vi "GetAlazar_SaveToFile_25_AVG.vi"(0 "AlazarCluster":T5, 1 "Digitizer Settings":T1={"Digitizer delay (us) "=0.0, "rf points per line"=2048, "lines per plane"=128, "Samp Rate (Hz)"=100000000.0, "Additional dig delay (us)"=0.0, "Voltage Scale"=0.4, "Pre-Looks"=0, "Offset delay (us)"=0.0, "bits A/D"=8, "Avg Num"=1, "DigTimeOut"=5.0, "Rel Dig Delay"=0.0, "Dig Ch"=0, "LeCroyCluster"={"LeCroy Channels"=[TRUE, FALSE, FALSE, FALSE], "LC read pt offset"=0.0, "Sweep Avg"=FALSE}, "Main Digitizer"=enum."NI Digitizer", "Dig Config"=enum."Single channel", "Digitizer ID Cluster"={"Acqiris/Alazar/SP ID"=[], "NI Instr Handles"=[], "LeCroy VISA"="", "GaGe Handle"={"Handle"=0, "Sample size"=0, "Resolution"=0, "Offset"=0, "Channels"=0, "Boards"=0}, "ATS Ref"="ATS9350", "Acqiris Address"=["PCI::INSTR0"], "ADQRef"=refnum, "adq_cu_ptr"=refnum}, "Trigger Settings"={"Trig Source"=1, "Trig Coupling"=0, "Trig Slope"=0, "Level (mV)"=1500.0}, "Bulk Acq"=FALSE, "Bulk Start Indexes"=[], "Data Ref RF"=refnum, "NI ID/Channel"=[], "Total Dig CH"=1, "Xtra Ann Trig delay (us)"=10.0, "Fix Z Delay?"=FALSE, "One Way Transmission?"=FALSE, "Data Ref Log"=refnum} {"Trigger Settings"."Trig Slope" items=["Positive", "Negative"]; "Trigger Settings"."Level (mV)" format="%.2f"; "Trigger Settings"."Trig Coupling" items=["DC 1 MOhm", "AC 1 MOhm", "DC 50 Ohm", "AC 50 Ohm"]; "Trigger Settings"."Trig Source" items=["Chan 1", "External"]; "Rel Dig Delay" format="%.2f"; "DigTimeOut" format="%.2f"; "Avg Num" min=1; "Offset delay (us)" format="%.2f"; "Additional dig delay (us)" format="%.2f"; "Digitizer delay (us)" format="%.2f"}, 7 "errorin":errorcluster, 8 "File Array":string[](array[string]), 10 "lines per plane":i32) -> (17 "Raw VGain (scale)":dbl, 18 "Gain Array":T6(array[cluster]), 20 "data out":i16[][][](array[numeric]), 21 "VGain (dB)":dbl, 27 "error out":errorcluster)   [LabVIEW 2022 SP3]
uses:
  -DigitizerRoutines/DigitizerSettings.ctl
  -DigitizerRoutines/DigitizerID.ctl
  -DigitizerRoutines/Digitizer.ctl
  -DigitizerRoutines/DigConfig.ctl
  C:/Windows/System32/ADQAPI_dotNet_helper.dll
panel:
  out "read time":u32
  out "save time":u32
  out "Numeric":i32
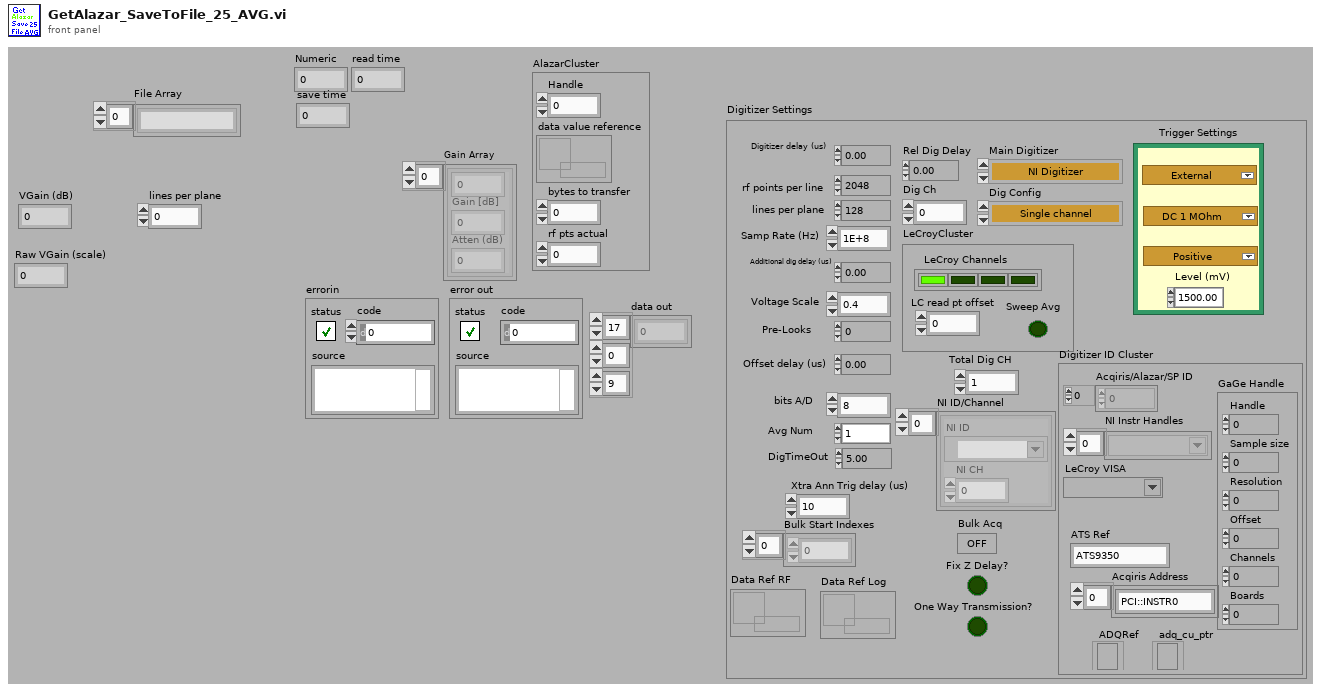
[diagram p1: front panel]
types:
  T1 = typedef "DigitizerSettings.ctl" = cluster{"Digitizer delay (us) ":dbl, "rf points per line":i32, "lines per plane":i32, "Samp Rate (Hz)":dbl, "Additional dig delay (us)":dbl, "Voltage Scale":dbl, "Pre-Looks":i32, "Offset delay (us)":dbl, "bits A/D":i8, "Avg Num":i32, "DigTimeOut":sgl, "Rel Dig Delay":sgl, "Dig Ch":i32, "LeCroyCluster":cluster{"LeCroy Channels":bool[], "LC read pt offset":dbl, "Sweep Avg":bool}, "Main Digitizer":T2, "Dig Config":T3, "Digitizer ID Cluster":T4, "Trigger Settings":cluster{"Trig Source":u16, "Trig Coupling":u16, "Trig Slope":u16, "Level (mV)":dbl}, "Bulk Acq":bool, "Bulk Start Indexes":i32[], "Data Ref RF":refnum<data-value>, "NI ID/Channel":cluster{"NI ID":refnum<k15>, "NI CH":i32}[], "Total Dig CH":i32, "Xtra Ann Trig delay (us)":dbl, "Fix Z Delay?":bool, "One Way Transmission?":bool, "Data Ref Log":refnum<data-value>}
  T2 = typedef "Digitizer.ctl" = enum16{"Acqiris Digitizer", "NI Digitizer", "LeCroy", "GaGe", "AlazarTech", "No Digitizer", "Teledyne"}
  T3 = typedef "DigConfig.ctl" = enum16{"Single channel", "2 Chans w/ 2 Acqiris", "2 Chans w/ 1 Acqiris", "5-CH Pulser New", "5-CH pulser w/ ann array", "5-pass style ann array", "Empty"}
  T4 = typedef "DigitizerID.ctl" = cluster{"Acqiris/Alazar/SP ID":u32[], "NI Instr Handles":refnum<k15>[], "LeCroy VISA":refnum<visa-resource-name>, "GaGe Handle":cluster{"Handle":u32, "Sample size":u32, "Resolution":i32, "Offset":i32, "Channels":u32, "Boards":u32}, "ATS Ref":string, "Acqiris Address":string[], "ADQRef":refnum<k24>, "adq_cu_ptr":refnum<k24>}
  T5 = cluster{"Handle":u32, "data value reference":refnum<data-value>, "bytes to transfer":u32, "rf pts actual":u32}
  T6 = cluster{sgl, "Gain [dB]  ":sgl, "Atten (dB)":sgl}[]
  T7 = cluster{"wfm":i16[][], "max queue size (-1, unlimited)":i32}
  T8 = cluster{sgl, "Gain [dB]  ":sgl, "Atten (dB)":sgl}
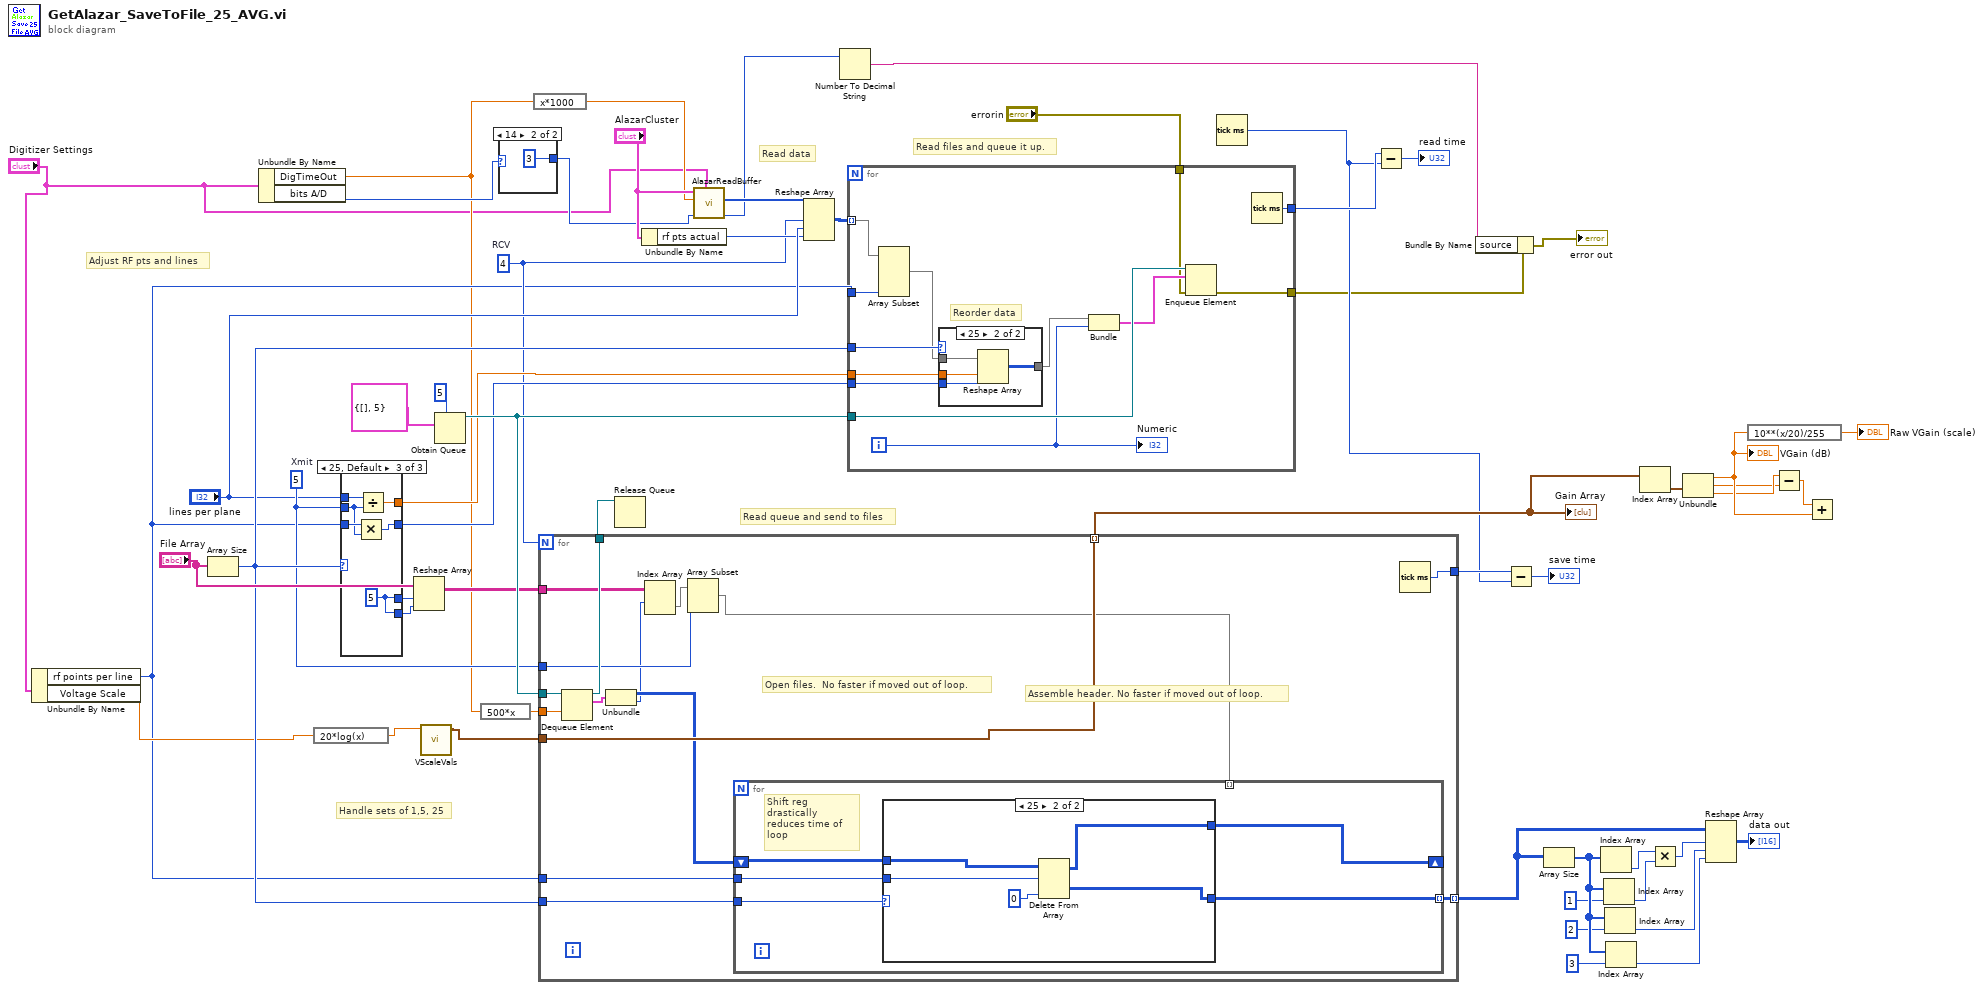
[diagram p0: block diagram]
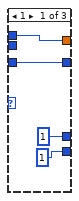
[diagram p4: hidden frame]
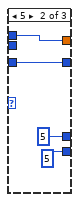
[diagram p5: hidden frame]
diagram:
  w30 = 5  # Xmit
  w24 = 4  # RCV
  # "Read data"
  # "Adjust RF pts and lines"
  # "Handle sets of 1,5, 25"
  # "Read files and queue it up."
  # "Read queue and send to files"
  n1 = Unbundle By Name("Digitizer Settings") -> ("rf points per line"=w4:i32, "Voltage Scale"=w5:dbl)
  n2 = Array Size(array="File Array") -> (size(s)=w34:i32)
  n3 = Unbundle By Name("Digitizer Settings") -> ("DigTimeOut"=w2:sgl, "bits A/D"=w3:i8)
  n4 = expression code="20*log(x)"(w5) -> (w32:dbl)
  n5 = case shown="25, Default" w34 {
    tunnel: [1 5 w70] -> w39
    tunnel: [w59 w63 w66] -> w36
    tunnel: w4 -> [w59 w63 w67]
    tunnel: [w58 w62 w68] -> w37
    tunnel: "lines per plane" -> [w58 w62 w69]
    tunnel: [1 5 w70] -> w38
    tunnel: w30 -> [_ _ w65]
    frame 1 {
    }
    frame 5 {
    }
    frame 25, Default {
      w70 = 5
      n6 = Multiply(x=w67, y=w65) -> (x*y=w66:i32)
      n7 = Divide(x=w69, y=w65) -> (x/y=w68:dbl)
    }
  }
  n8 = Reshape Array("File Array", w39, w38) -> (w33:string[][])
  n9 = call "VScaleVals.vi"("Full Scale"=w32) -> ("Voltage Scale"=w31:T8)  [unwired: 8 in, 2 out]
  n10 = Obtain Queue(max queue size (-1, unlimited)=5, element data type=T7 {"wfm"=[], "max queue size (-1, unlimited)"=5}) -> (queue out=w48:refnum<queue>)  [unwired: 3 in, 2 out]
  n11 = expression code="500*x"(w2) -> (w35:sgl)
  n12 = case shown="14" w3 {
    tunnel: [_ u16 3 ("Extra Shift")] -> w17
    frame 0, Default {
    }
    frame 14 {
    }
  }
  n13 = expression code="x*1000"(w2) -> (w22:sgl)
  n14 = for {
    N: w24 -> [_]
    tunnel: w4 -> [w86]
    tunnel: [w76] -> w49 mode=indexing
    tunnel: w48 -> [w85]
    tunnel: [w83] -> w41
    tunnel: [w82] -> w45
    tunnel: w34 -> [w81]
    tunnel: w35 -> [w80]
    tunnel: w33 -> [w79]
    tunnel: w30 -> [w77]
    tunnel: w31 -> [w76]
    tunnel: [w73] -> w6 mode=indexing
    # "Open files.  No faster if moved out of loop."
    # "Assemble header. No faster if moved out of loop."
    n15 = Dequeue Element(queue=w85, timeout in ms (-1)=w80) -> (queue out=w83:refnum<queue>, element=w84:T7)  [unwired: 1 in, 2 out]
    n16 = Unbundle(w84) -> ("wfm"=w75:i16[][], "max queue size (-1, unlimited)"=w74:i32)
    n17 = Index Array(array=w79, index (row)=w74) -> (element=w78:string[])  [unwired: 1 in]
    n18 = Array Subset(array=w78, length=w77) -> (w72:string[])  [unwired: 1 in]
    n19 = for {
      tunnel: w72 -> [_] mode=indexing
      tunnel: w86 -> [w91]
      tunnel: w81 -> [w89]
      shift-right: [w88] -> _
      shift-left: w75 -> [w90]
      tunnel: [w87] -> w73 mode=indexing
      # "Shift reg drastically reduces time of loop"
      n20 = case shown="25" w89 {
        tunnel: w91 -> [_ w95]
        tunnel: w90 -> [w92 w97]
        tunnel: [w92 w96] -> w88
        tunnel: [w92 w93] -> w87
        frame 5, Default {
        }
        frame 25 {
          n21 = Delete From Array(array=w97, length=w95, index (col)=0 ("index (row)")) -> (deleted portion=w93:i16[][], array with subset deleted=w96:i16[][])  [unwired: 1 in]
        }
      }
    }
    n22 = Tick Count (ms)() -> (millisecond timer value=w82:u32)
  }
  "Gain Array" <- w49
  n23 = Release Queue(queue=w41) -> ()  [unwired: 2 in, 3 out]
  n24 = Unbundle By Name("AlazarCluster") -> ("rf pts actual"=w26:u32)
  n25 = call "AlazarReadBuffer.vi"("Digitizer Settings"="Digitizer Settings", "Extra Shift"=w17, "time out"=w22, "AlazarCluster"="AlazarCluster") -> ("Return Code"=w18:u32, "Data Array"=w27:i16[])  [unwired: 5 in, 1 out]
  n26 = Reshape Array(w27, w24, "lines per plane", w26) -> (w25:i16[][][])
  n27 = Number To Decimal String(number=w18) -> (decimal integer string=w20:string)  [unwired: 1 in]
  n28 = for {
    tunnel: w48 -> [w110]
    tunnel: [w108] -> w46
    tunnel: [w107] -> w21
    tunnel: w34 -> [w106]
    tunnel: w37 -> [w105]
    tunnel: w36 -> [w104]
    tunnel: w25 -> [w102] mode=indexing
    tunnel: w4 -> [w101]
    tunnel: "errorin" -> [w98]
    i -> [w99]
    # "Reorder data"
    n29 = Array Subset(array=w102, length (col)=w101) -> (w100:i16[][])  [unwired: 3 in]
    n30 = case shown="25" w106 {
      tunnel: w104 -> [_ w115]
      tunnel: w100 -> [w111 w114]
      tunnel: [w111 w113] -> w103
      tunnel: w105 -> [_ w112]
      frame 0, Default {
      }
      frame 25 {
        n31 = Reshape Array(w114, w112, w115) -> (w113:i16[][])
      }
    }
    n32 = Bundle(w103, w99) -> (w109:cluster{i16[][], i32})  [unwired: 1 in]
    n33 = Enqueue Element(queue=w110, element=w109, error in (no error)=w98) -> (error out=w107:errorcluster)  [unwired: 1 in, 2 out]
    n34 = Tick Count (ms)() -> (millisecond timer value=w108:u32)
    "Numeric" <- w99
  }
  n35 = Tick Count (ms)() -> (millisecond timer value=w44:u32)
  n36 = Subtract(x=w46, y=w44) -> (x-y=→"read time":u32)
  n37 = Bundle By Name(cluster=w21, "source"=w20) -> (→"error out":errorcluster)
  n38 = Subtract(x=w45, y=w44) -> (x-y=→"save time":u32)
  n39 = Array Size(array=w6) -> (size(s)=w16:i32[])
  n40 = Index Array(array=w16) -> (element=w12:i32)  [unwired: 1 in]
  n41 = Index Array(array=w16, index=1) -> (element=w13:i32)
  n42 = Index Array(array=w16, index=2) -> (element=w15:i32)
  n43 = Index Array(array=w16, index=3) -> (element=w14:i32)
  n44 = Index Array(array=w49) -> (element=w56:T8)  [unwired: 1 in]
  n45 = Multiply(x=w12, y=w13) -> (x*y=w11:i32)
  n46 = Unbundle(w56) -> (w55:sgl, "Gain [dB]"=w53:sgl, "Atten (dB)"=w54:sgl)
  "VGain (dB)" <- w55
  n47 = Reshape Array(w6, w11, w15, w14) -> (→"data out":i16[][][])
  n48 = expression code="10**(x/20)/255"(w55) -> (→"Raw VGain (scale)":sgl)
  n49 = Subtract(x=w54, y=w53) -> (x-y=w52:sgl)
  n50 = Add(x=w52, y=w55) -> ()  [unwired: 1 out]
